vi "read exception property.vi"   [LabVIEW 2013]
doc: "This VI is used to read data stored in a Variant Repository, similar to a look up table. This VI is will get an attribute of the <b>Variant Repository In</b>, with the tag name of <b>Tag</b>, and return its value on <b>Value</b>, and then return the same varient data on <b>Varient Repository Out</b>. This VI will put an error on the <b>error out</b> if the tag is not found, there is no tag when needed, or the tag was found, but of the wrong data type.\n\nRight click and Select Type for simple data types, or choose Automatic and wire in the <b>Data Type</b> to be read.\n\nIf the a data type is selected, then the <b>Tag</b> must also be provided. If the data type is selected using the <b>Data Type</b> input then the tag is optional, and if empty the label associated with the data passed in will be used as the tag.\n\nReading multiple tags can be done by right clicking and choosing Read Multiple Tags.\n\n-------------\nBrian Hoover (Hooovahh)\n\nProduct Name: Variant Repository\nPackage File Name: lava_lib_variant_repository\nPackage Version: 1.0.1.11\nMinimum LabVIEW Version: 11.0"
uses:
  severity.ctl
  exception.lvlib
  category.ctl
  exception.ctl
  Read Variant Repository/Read Exception Property.xnode
  <vilib>/Utility/VariantDataType/GetTypeInfo.vi
  <vilib>/Utility/VariantDataType/VariantType.lvlib
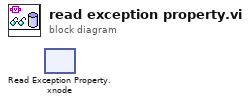
[diagram p0: block diagram]
diagram:
  n1 = xnode "Read Exception Property.xnode"() -> ()  [unwired: 3 in, 3 out]
